vi "Simple Queue.vi"() -> ()   [LabVIEW 2023]
doc: "This VI creates two queues to pass data between parallel loops. Queues are most useful when you need to send data from one or more data sources to one data sink with no potential loss of data."
panel:
  out "Data 2":dbl(graph)
  out "Data 1":dbl(graph)
  in  "Stop":bool
  # "Overview: Demonstrates the use of the Queue functions to pass data between parallel loops.\nInstructions:\nRun the VI."
  # "The data generated by Loop 1 on the diagram is passed to Loop 2 through a queue. The stop condition is also monitored in Loop 1 and sent to Loop 2 in a queue."
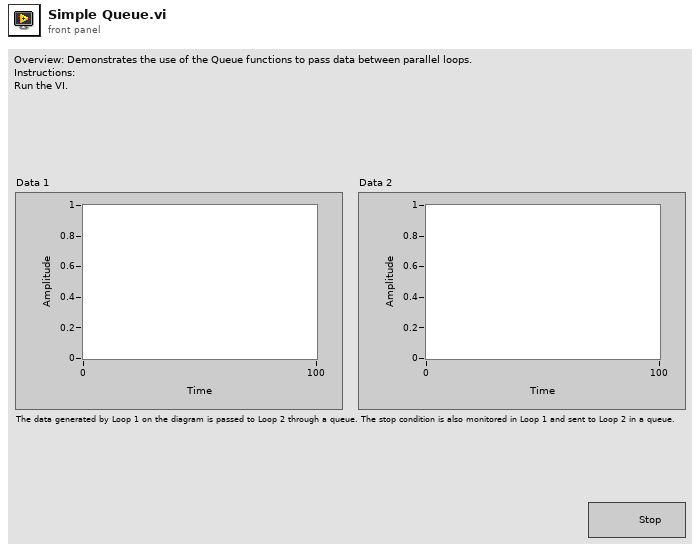
[diagram p1: front panel]
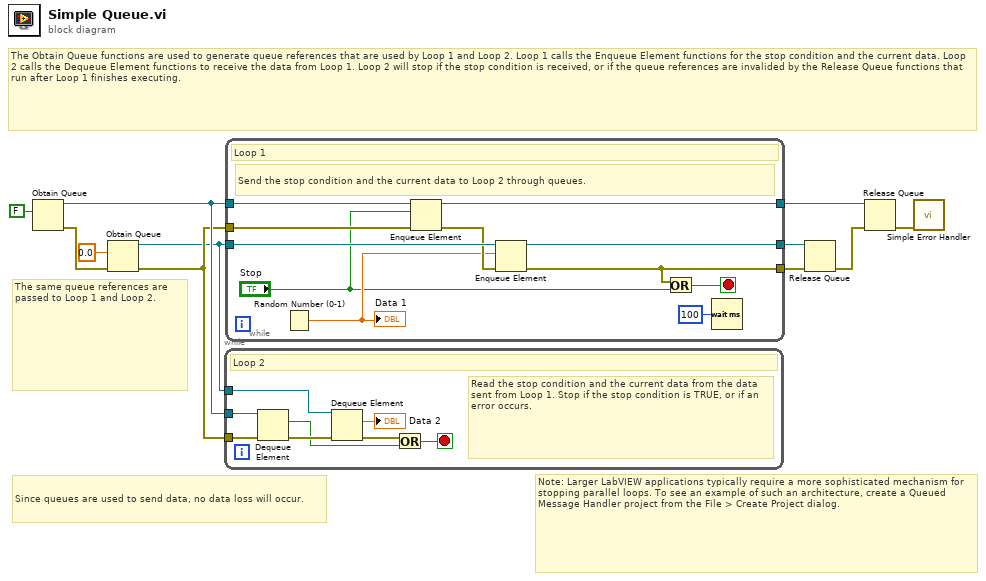
[diagram p0: block diagram]
diagram:
  # "Since queues are used to send data, no data loss will occur."
  # "Note: Larger LabVIEW applications typically require a more sophisticated mechanism for stopping parallel loops. To see an example of such an architecture, create a Queued Message Handler project from the File > Create Project dialog."
  # "The same queue references are passed to Loop 1 and Loop 2."
  # "The Obtain Queue functions are used to generate queue references that are used by Loop 1 and Loop 2. Loop 1 calls the Enqueue Element functions for the stop condition and the current data. Loop 2 calls the Dequeue Element functions to receive the data from Loop 1. Loop 2 will stop if the stop condition is received, or if the queue references are invalided by the Release Queue functions that run after Loop 1 finishes executing."
  n1 = Obtain Queue(element data type=FALSE) -> (queue out=w11:refnum<queue>, error out=w9:errorcluster)  [unwired: 4 in, 1 out]
  n2 = Obtain Queue(element data type=0.0, error in (no error)=w9) -> (queue out=w1:refnum<queue>, error out=w2:errorcluster)  [unwired: 3 in, 1 out]
  n3 = while {
    tunnel: w11 -> [w18]
    tunnel: w2 -> [w19]
    tunnel: w1 -> [w16]
    stop <- w12 stop-if-true
    # "Read the stop condition and the current data from the data sent from Loop 1. Stop if the stop condition is TRUE, or if an error occurs."
    # "Loop 2"
    n4 = Dequeue Element(queue=w18, error in (no error)=w19) -> (element=w13:bool, error out=w17:errorcluster)  [unwired: 1 in, 2 out]
    n5 = Dequeue Element(queue=w16, error in (no error)=w17) -> (element=→"Data 2":dbl, error out=w14:errorcluster)  [unwired: 1 in, 2 out]
    n6 = Or(x=w14, y=w13) -> (x .or. y?=w12:bool)
  }
  n7 = while {
    tunnel: w11 -> [w29]
    tunnel: w2 -> [w28]
    tunnel: [w27] -> w4
    tunnel: w1 -> [w26]
    tunnel: [w24] -> w6
    tunnel: [w22] -> w7
    stop <- w20 stop-if-true
    # "Send the stop condition and the current data to Loop 2 through queues."
    # "Loop 1"
    n8 = Random Number (0-1)() -> (number: 0 to 1=w23:dbl)
    "Data 1" <- w23
    n9 = Enqueue Element(queue=w29, element="Stop", error in (no error)=w28) -> (queue out=w27:refnum<queue>, error out=w25:errorcluster)  [unwired: 1 in, 1 out]
    n10 = Enqueue Element(queue=w26, element=w23, error in (no error)=w25) -> (queue out=w24:refnum<queue>, error out=w22:errorcluster)  [unwired: 1 in, 1 out]
    n11 = Or(x=w22, y="Stop") -> (x .or. y?=w20:bool)
    n12 = Wait (ms)(milliseconds to wait=u32 100) -> ()  [unwired: 1 out]
  }
  n13 = Release Queue(queue=w6, error in (no error)=w7) -> (error out=w5:errorcluster)  [unwired: 1 in, 2 out]
  n14 = Release Queue(queue=w4, error in (no error)=w5) -> (error out=w3:errorcluster)  [unwired: 1 in, 2 out]
  n15 = call <vilib>:"Simple Error Handler.vi"("error in (no error)"=w3) -> ()  [unwired: 4 in, 5 out]
